vi "1D Linear Evaluation PtByPt.vi"(1 "offset":dbl format="%0.2f", 2 "scale":dbl format="%0.2f", 3 "x":dbl format="%0.2f") -> (0 "y[i]=x[i]*a+b":dbl format="%0.2f")   [LabVIEW 2020, in "NI_PtbyPt.lvlib"]
doc: "Performs a linear evaluation of <B>x</B>."
uses:
  NI_PtbyPt.lvlib
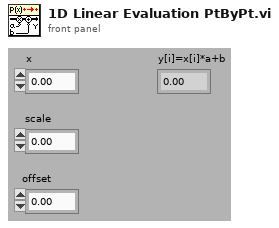
[diagram p1: front panel]
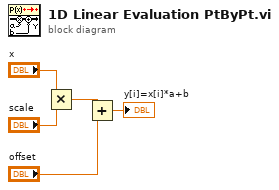
[diagram p0: block diagram]
diagram:
  n1 = Multiply(x="x", y="scale") -> (x*y=w3:dbl)
  n2 = Add(x=w3, y="offset") -> (x+y=→"y[i]=x[i]*a+b":dbl)
